vi "WPI_PWMGetValue.vi"(8 "error in (no error)":errorcluster, 11 "PWMDeviceRef":T1={"DeviceStatus"={"status"=FALSE, "code"=0, "source"=""}, "PWM Channel"=enum."PWM 4"}) -> (0 "error out":errorcluster, 2 "Value":u8, 3 "PWMDeviceRef":T1={"DeviceStatus"={"status"=FALSE, "code"=0, "source"=""}, "PWM Channel"=enum."PWM 4"})   [LabVIEW 2017]
doc: "Returns the raw value from the PWM you specify. The raw PWM value ranges from 0 to 255. A value of 1 puts the motor controller in full reverse, a value of 255 puts the motor controller in full forward, and a value of 0 disables the motor controller. Use this VI with custom motor controllers. Use the GetSpeed VI on the MotorControl palette to return PWM values from the Jaguar or Victor motor controllers.\n\nThis software is licensed. Open the labview\\readme\\WPI Robotics Library Open Source License.txt file for more information."
uses:
  <vilib>/Rock Robotics/WPI/PWM/WPI_PWMDeviceRef.ctl
  <vilib>/Rock Robotics/SystemInterfaces/DIO/FPGA_DIOPWMChannel.ctl
  <vilib>/Rock Robotics/WPI/PWM/WPI_PWMChannelCacheOp.ctl
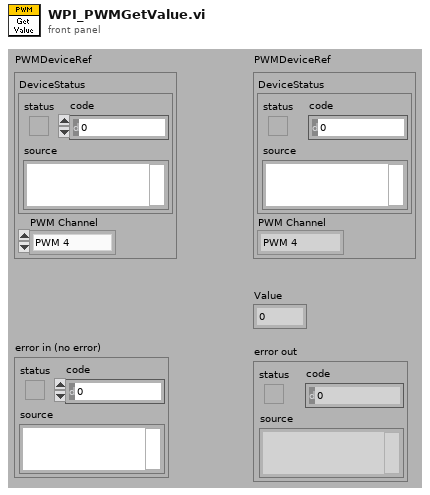
[diagram p1: front panel]
types:
  T1 = typedef "WPI_PWMDeviceRef.ctl" = cluster{"DeviceStatus":errorcluster, "PWM Channel":T2}
  T2 = typedef "FPGA_DIOPWMChannel.ctl" = enum8{"PWM 0", "PWM 1", "PWM 2", "PWM 3", "PWM 4", "PWM 5", "PWM 6", "PWM 7", "PWM 8", "PWM 9", "PWM MXP 0", "PWM MXP 1", "PWM MXP 2", "PWM MXP 3", "PWM MXP 4", "PWM MXP 5", "PWM MXP 6", "PWM MXP 7", "PWM MXP 8", "PWM MXP 9", "Invalid"}
  T3 = typedef "WPI_PWMChannelCacheOp.ctl" = enum16{"Acquire", "Release", "Status"}
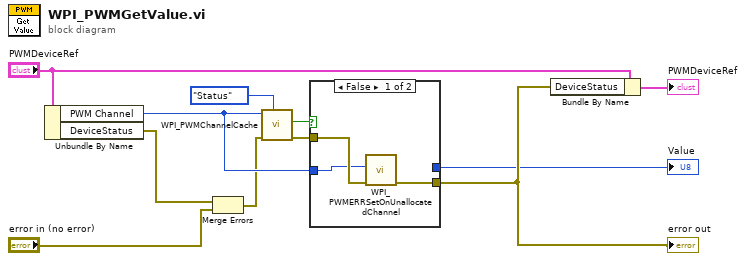
[diagram p0: block diagram]
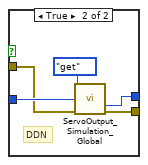
[diagram p2: hidden frame]
diagram:
  n1 = Unbundle By Name("PWMDeviceRef") -> ("PWM Channel"=w4:T2, "DeviceStatus"=w2:errorcluster)
  n2 = Merge Errors(w2, "error in (no error)") -> (w1:errorcluster)
  n3 = call <vilib>:"WPI_PWMChannelCache.vi"("Operation"=WPI_PWMChannelCacheOp."Status", "error in (no error)"=w1, "PWMChannel"=w4) -> ("error out"=w5:errorcluster, "Allocated?"=w6:bool)  [unwired: 2 in, 5 out]
  n4 = case shown="False" w6 {
    tunnel: [_ w17] -> w8
    tunnel: [w13 w18] -> w10
    tunnel: w5 -> [w14 w15]
    tunnel: w4 -> [w12 w16]
    frame False {
      n5 = call <vilib>:"WPI_PWMERRSetOnUnallocatedChannel.vi"("error in (no error)"=w14, "PWM Channel"=w12) -> ("error out"=w13:errorcluster)  [unwired: 9 in]
    }
    frame True {
      # "DDN"
      n6 = call <vilib>:"ServoOutput_Simulation_Global.vi"("menu"=enum16{"set", "get", "delete"}."get", "PWM Channel"=w16, "error in (no error)"=w15) -> ("Output Get"=w17:u8, "error out"=w18:errorcluster)  [unwired: 11 in]
    }
  }
  "Value" <- w8
  "error out" <- w10
  n7 = Bundle By Name(cluster="PWMDeviceRef", "DeviceStatus"=w10) -> (→"PWMDeviceRef":T1)
